vi "Random element (SubVI).vi"(11 "Array":i32[](array[numeric])) -> (3 "random element":i32)   [LabVIEW 2013]
doc: "Randomly returns an element from the input array."
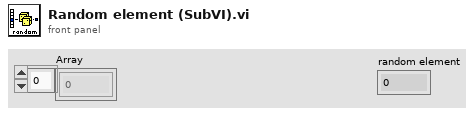
[diagram p1: front panel]
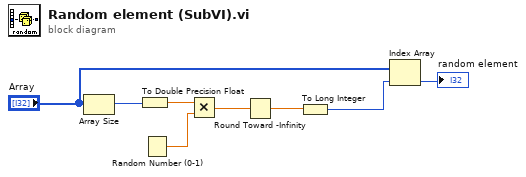
[diagram p0: block diagram]
diagram:
  n1 = Array Size(array="Array") -> (size(s)=w8:i32)
  n2 = To Double Precision Float(number=w8) -> (double precision float=w5:dbl)
  n3 = Random Number (0-1)() -> (number: 0 to 1=w7:dbl)
  n4 = Multiply(x=w5, y=w7) -> (x*y=w6:dbl)
  n5 = Round Toward -Infinity(1:w6) -> (0:w4:dbl)
  n6 = To Long Integer(number=w4) -> (32bit integer=w2:i32)
  n7 = Index Array(array="Array", index=w2) -> (element=→"random element":i32)
